vi "Test Data.vi"(8 "error in (no error)":errorcluster, 11 "Instrument.Lockin in":refnum<class "Instrument.Lockin.lvclass">) -> (0 "error out":errorcluster, 3 "Instrument.Lockin out":refnum<class "Instrument.Lockin.lvclass">)   [LabVIEW 2016]
uses:
  src/Instrument.Lockin/Instrument.Lockin.lvclass
  <vilib>/addons/_JKI Toolkits/Caraya/classes/Assert/Assert Not Error.vi
  <vilib>/addons/_JKI Toolkits/Caraya/classes/Assert/Assert False.vi
  <vilib>/addons/_JKI Toolkits/Caraya/classes/Test/Test.lvclass
  <vilib>/addons/_JKI Toolkits/Caraya/classes/Assert/Assert.lvclass
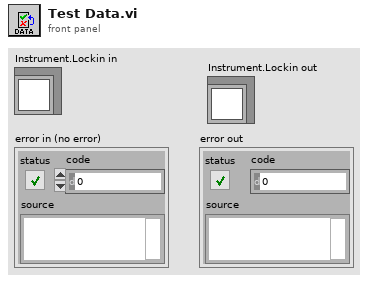
[diagram p1: front panel]
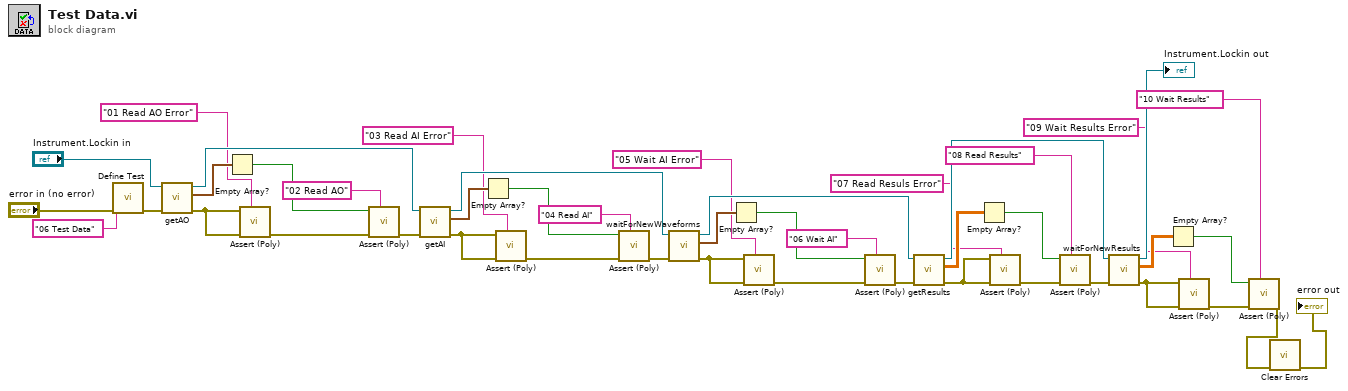
[diagram p0: block diagram]
diagram:
  n1 = call <vilib>:"Define Test.vi"("error in (no error)"="error in (no error)", "Label (VI Title)"="06 Test Data") -> ("error out"=w38:errorcluster)  [unwired: 9 in]
  n2 = call "getAO.vi"("error in (no error)"=w38, "Instrument.Lockin in"="Instrument.Lockin in") -> ("error out"=w37:errorcluster, "AO Waveforrm"=w32:waveform(dbl)[], "Instrument.Lockin out"=w42:refnum<class "Instrument.Lockin.lvclass">)  [unwired: 7 in]
  n3 = Empty Array?(array=w32) -> (empty?=w31:bool)
  n4 = call-poly <vilib>:"Assert (Poly).vi"("Label"="01 Read AO Error", "error in (no error)"=w37, "Not Error?"=w37) -> ("error out"=w30:errorcluster)  [unwired: 8 in]
  n5 = call-poly <vilib>:"Assert (Poly).vi"("Label"="02 Read AO", "error in (no error)"=w30, "False?"=w31) -> ("error out"=w23:errorcluster)  [unwired: 8 in]
  n6 = call "getAI.vi"("error in (no error)"=w23, "Instrument.Lockin in"=w42) -> ("error out"=w36:errorcluster, "AI Waveform"=w29:waveform(dbl)[], "Instrument.Lockin out"=w43:refnum<class "Instrument.Lockin.lvclass">)  [unwired: 7 in]
  n7 = Empty Array?(array=w29) -> (empty?=w28:bool)
  n8 = call-poly <vilib>:"Assert (Poly).vi"("Label"="03 Read AI Error", "error in (no error)"=w36, "Not Error?"=w36) -> ("error out"=w24:errorcluster)  [unwired: 8 in]
  n9 = call-poly <vilib>:"Assert (Poly).vi"("Label"="04 Read AI", "error in (no error)"=w24, "False?"=w28) -> ("error out"=w22:errorcluster)  [unwired: 8 in]
  n10 = call "waitForNewWaveforms.vi"("error in (no error)"=w22, "Instrument.Lockin in"=w43) -> ("error out"=w35:errorcluster, "Newest AI Waveform"=w27:waveform(dbl)[], "Instrument.Lockin out"=w44:refnum<class "Instrument.Lockin.lvclass">)  [unwired: 7 in]
  n11 = Empty Array?(array=w27) -> (empty?=w26:bool)
  n12 = call-poly <vilib>:"Assert (Poly).vi"("Label"="05 Wait AI Error", "error in (no error)"=w35, "Not Error?"=w35) -> ("error out"=w25:errorcluster)  [unwired: 8 in]
  n13 = call-poly <vilib>:"Assert (Poly).vi"("Label"="06 Wait AI", "error in (no error)"=w25, "False?"=w26) -> ("error out"=w21:errorcluster)  [unwired: 8 in]
  n14 = call "getResults.vi"("error in (no error)"=w21, "Instrument.Lockin in"=w44) -> ("error out"=w34:errorcluster, "Results"=w20:dbl[][], "Instrument.Lockin out"=w45:refnum<class "Instrument.Lockin.lvclass">)  [unwired: 6 in, 1 out]
  n15 = Empty Array?(array=w20) -> (empty?=w19:bool)
  n16 = call-poly <vilib>:"Assert (Poly).vi"("Label"="07 Read Resuls Error", "error in (no error)"=w34, "Not Error?"=w34) -> ("error out"=w18:errorcluster)  [unwired: 8 in]
  n17 = call-poly <vilib>:"Assert (Poly).vi"("Label"="08 Read Results", "error in (no error)"=w18, "False?"=w19) -> ("error out"=w14:errorcluster)  [unwired: 8 in]
  n18 = call "waitForNewResults.vi"("error in (no error)"=w14, "Instrument.Lockin in"=w45) -> ("error out"=w33:errorcluster, "Results"=w17:dbl[][], "Instrument.Lockin out"=→"Instrument.Lockin out":refnum<class "Instrument.Lockin.lvclass">)  [unwired: 7 in]
  n19 = Empty Array?(array=w17) -> (empty?=w16:bool)
  n20 = call-poly <vilib>:"Assert (Poly).vi"("Label"="09 Wait Results Error", "error in (no error)"=w33, "Not Error?"=w33) -> ("error out"=w15:errorcluster)  [unwired: 8 in]
  n21 = call-poly <vilib>:"Assert (Poly).vi"("Label"="10 Wait Results", "error in (no error)"=w15, "False?"=w16) -> ("error out"=w3:errorcluster)  [unwired: 8 in]
  n22 = call <vilib>:"Clear Errors.vi"("error in (no error)"=w3) -> ("error out"=→"error out":errorcluster)  [unwired: 5 in, 1 out]
